vi "script - Copy.vi"() -> ()   [LabVIEW 2016]
panel:
  out "VI Name 2":string
  in  "error in (no error)":errorcluster
  out "Application:All VIs In Memory 2":string[](array[string])
  out "VI Name":string
  out "appended array":errorcluster[](array[cluster])
  out "Application:All VIs In Memory":string[](array[string])
  out "error out":errorcluster
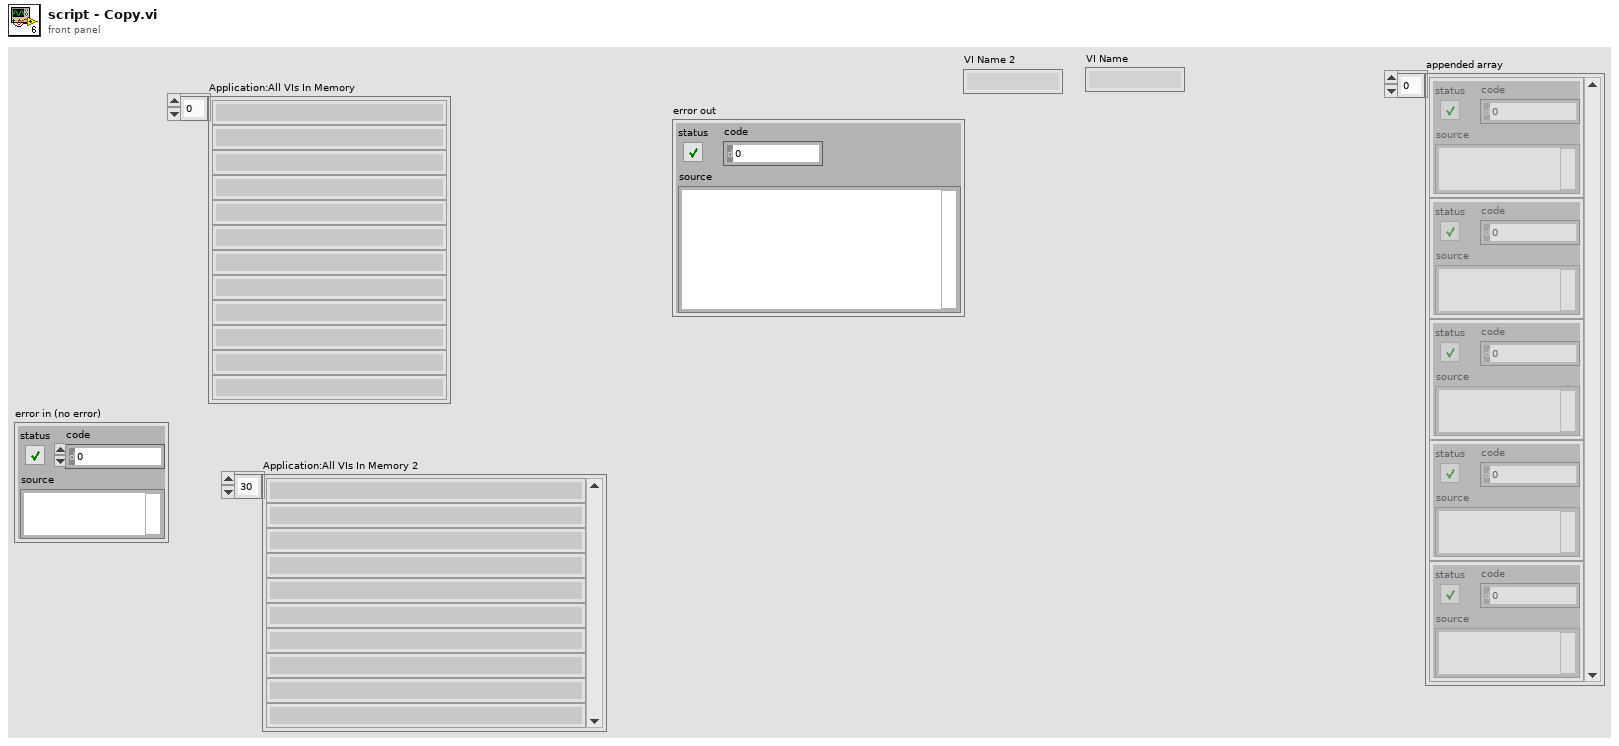
[diagram p1: front panel]
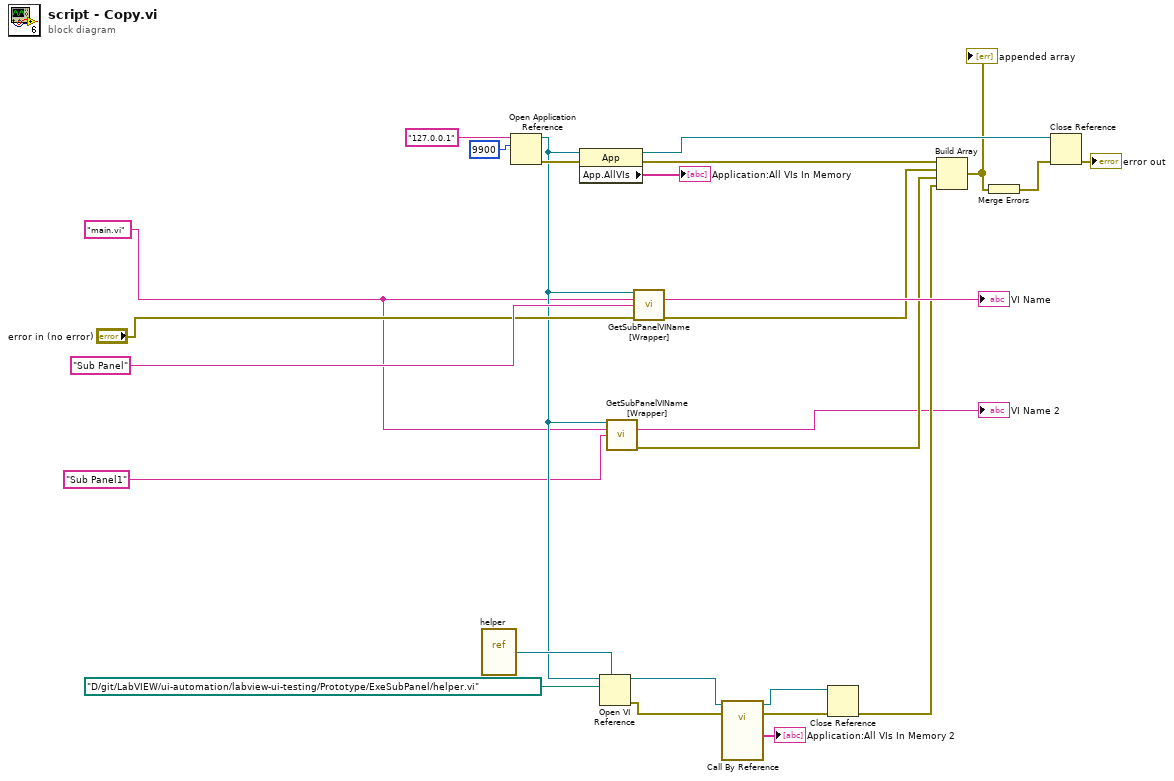
[diagram p0: block diagram]
diagram:
  w3 = "main.vi" ("y")
  n1 = vi-ref "helper.vi"() -> (w14:refnum<vi>)
  n2 = Open Application Reference(10:u16 9900 ("port number or service name (3363)"), 11:"127.0.0.1" ("machine name (\"\":  open local reference)")) -> (0:w24:errorcluster, 3:w5:refnum<vi>)  [unwired: 2 in]
  n3 = property class="App"(reference=w5, error in=w24) -> (reference out=w23:refnum<vi>, error out=w18:errorcluster, "App.AllVIs"=→"Application:All VIs In Memory":string[])
  n4 = Open VI Reference(type specifier VI Refnum (for type only)=w14, application reference (local)=w5, vi path=path "D:/git/LabVIEW/ui-automation/labview-ui-testing/Prototype/ExeSubPanel/helper.vi") -> (vi reference=w13:refnum<vi>, error out=w12:errorcluster)  [unwired: 3 in]
  n5 = call "GetSubPanelVIName [Wrapper].vi"("Application in"=w5, "VI Name"=w3, "SubPanel Label"="Sub Panel1" ("y")) -> ("VI Name"=→"VI Name 2":string, "error out"=w2:errorcluster)  [unwired: 10 in, 1 out]
  n6 = call "GetSubPanelVIName [Wrapper].vi"("Application in"=w5, "VI Name"=w3, "SubPanel Label"="Sub Panel" ("y"), "error in (no error)"="error in (no error)") -> ("VI Name"=→"VI Name":string, "error out"=w6:errorcluster)  [unwired: 9 in, 1 out]
  n7 = call-by-ref "?"(reference=w13, error in=w12) -> (reference out=w10:refnum<vi>, error out=w11:errorcluster, "Application:All VIs In Memory"=→"Application:All VIs In Memory 2":string[])  [unwired: 10 in, 1 out]
  n8 = Close Reference(reference=w10, error in (no error)=w11) -> (error out=w8:errorcluster)
  n9 = Build Array(w18, w6, w2, w8) -> (w20:errorcluster[])
  "appended array" <- w20
  n10 = Merge Errors(w20) -> (w19:errorcluster)
  n11 = Close Reference(reference=w23, error in (no error)=w19) -> (error out=→"error out":errorcluster)
